vi "曲线查看.vi"(8 "曲线名":string[](array[string]), 11 "曲线数据":sgl[][](array[numeric])) -> (3 "前面板窗口:打开":bool)   [LabVIEW 2020]
panel:
  out "波形图":sgl[][](graph)
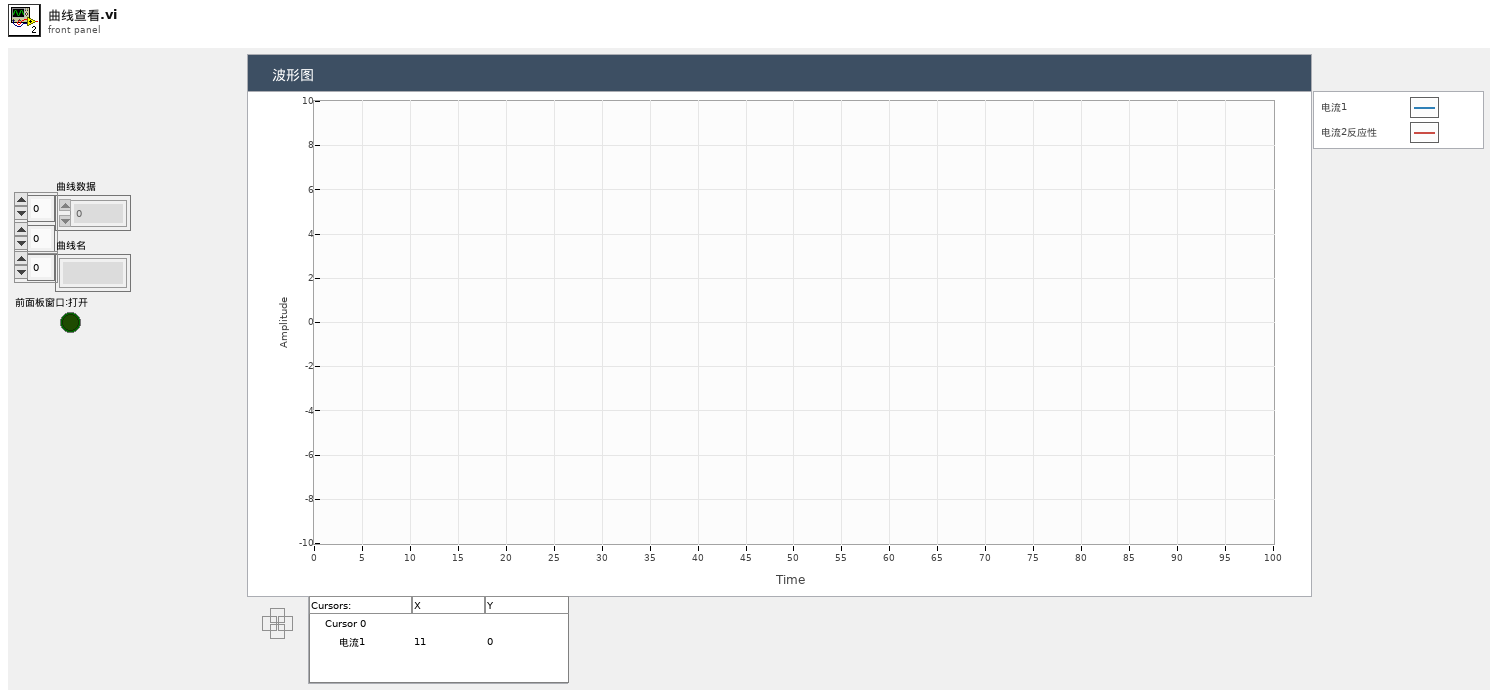
[diagram p1: front panel]
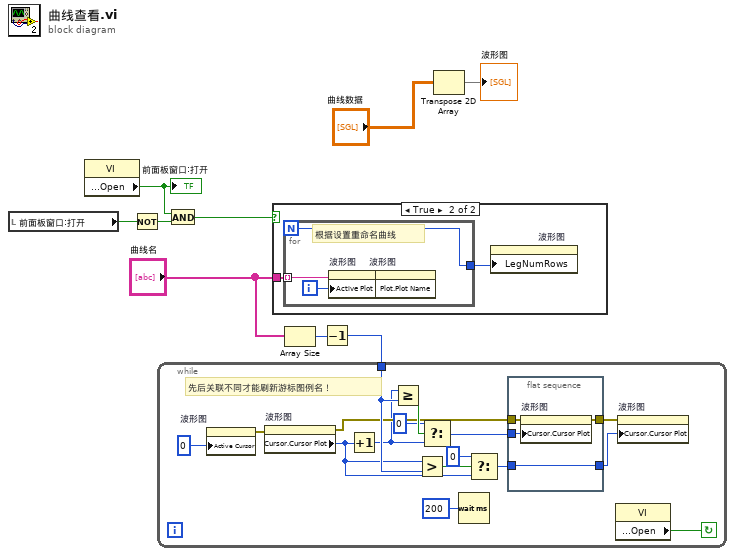
[diagram p0: block diagram]
diagram:
  n1 = local read "前面板窗口:打开"() -> (w5:bool)
  n2 = property class="VI"() -> ("Front Panel.Open"=w3:bool)  [unwired: 2 in, 2 out]
  "前面板窗口:打开" <- w3
  n3 = Not(x=w5) -> (.not. x?=w4:bool)
  n4 = And(x=w3, y=w4) -> (x .and. y?=w6:bool)
  n5 = case shown="True" w6 {
    tunnel: "曲线名" -> [_ w10]
    frame False {
    }
    frame True {
      n6 = for {
        N -> [w12]
        tunnel: w10 -> [w14] mode=indexing
        tunnel: [w12] -> w11
        i -> [w15]
        # "根据设置重命名曲线"
        n7 = property on="波形图" class="WFGraph (strict)"("Active Plot"=w15) -> (error out=w13:errorcluster)  [unwired: 2 in, 1 out]
        n8 = property on="波形图" class="WFGraph (strict)"(error in=w13, "Plot.Plot Name"=w14) -> ()  [unwired: 1 in, 2 out]
      }
      n9 = property on="波形图" class="WFGraph (strict)"("LegNumRows"=w11) -> ()  [unwired: 2 in, 2 out]
    }
  }
  n10 = Array Size(array="曲线名") -> (size(s)=w7:i32)
  n11 = Decrement(x=w7) -> (x-1=w9:i32)
  n12 = while {
    tunnel: w9 -> [w31]
    stop <- w17 continue-if-true
    # "先后关联不同才能刷新游标图例名！"
    n13 = property on="波形图" class="WFGraph (strict)"("Active Cursor"=u32 0 ("活动游标")) -> (error out=w30:errorcluster)  [unwired: 2 in, 1 out]
    n14 = property on="波形图" class="WFGraph (strict)"(error in=w30) -> (error out=w27:errorcluster, "Cursor.Cursor Plot"=w22:i32)  [unwired: 1 in, 1 out]
    n15 = Increment(x=w22) -> (x+1=w21:i32)
    n16 = Greater Or Equal?(x=w21, y=w31) -> (x >= y?=w29:bool)
    n17 = Greater?(x=w22, y=w31) -> (0:w24:bool)
    n18 = Select(t=0, s=w29, f=w21) -> (s? t:f=w26:i32)
    n19 = Wait (ms)(milliseconds to wait=u32 200 ("等待时间（毫秒）")) -> ()  [unwired: 1 out]
    n20 = Select(t=0, s=w24, f=w22) -> (s? t:f=w20:i32)
    n21 = flat-sequence {
      tunnel: [w35] -> w28
      tunnel: w27 -> [w34]
      tunnel: w26 -> [w33]
      tunnel: w20 -> [w32]
      tunnel: [w32] -> w19
      frame #0 {
        n22 = property on="波形图" class="WFGraph (strict)"(error in=w34, "Cursor.Cursor Plot"=w33) -> (error out=w35:errorcluster)  [unwired: 1 in, 1 out]
      }
    }
    n23 = property class="VI"() -> ("Front Panel.Open"=w17:bool)  [unwired: 2 in, 2 out]
    n24 = property on="波形图" class="WFGraph (strict)"(error in=w28, "Cursor.Cursor Plot"=w19) -> ()  [unwired: 1 in, 2 out]
  }
  n25 = Transpose 2D Array(2D array="曲线数据") -> (transposed array=→"波形图":sgl[][])
